vi "AcquisitionFastMode.vi"(10 "Data In":T1={"DAQ Config Data"={"Vertical"={"Coupling"=1, "Offset (V)"=-0.5, "Range (V)"=2.0, "Impedance"=50.0}, "Horizontal"={"Offset Time"=0.0, "Sample Time (S)"=22.0, "Sample Points"=1000}, "Trigger\n"={"Lower Level (V)"=-0.02, "Trigger Slope"=1, "Trigger Source"=10}, "Acquisition"={"Trigger Mode"=1, "Initiate Continuously"=0, "Acquire Type"=0, "Acquire Count"=0}, "Channel"=0, "Instrument Handle"=0, "Error"={"status"=FALSE, "code"=0, "source"=""}, "State"=1}, "Acquisition"={"Current"={"Acquiring Now?"=FALSE, "Waveforms Acquired"=0.0, "Start of Acquisition"=timestamp(0 s since 1904-01-01), "Acquisition Name"=""}, "Stop Condition"={"Quota"=3000.0, "Duration (S)"=22, "Stop Condition"=FALSE}, "Config Needed"=FALSE}, "Measurement"={"Waveform"={"t0"=timestamp(0 s since 1904-01-01), "dt"=1.0, "Y"=[]}, "Peak Heights"=[], "Acquisition Time"=timestamp(0 s since 1904-01-01), "File Path"=path "", "TDMS File Handle"=refnum}, "UI References"={"Acquire"=refnum, "Configure DAQ"=refnum, "Measurement (Ch1)"=refnum, "Update Needed?"=FALSE, "New Run"=refnum, "Signal"=refnum}, "Run Info"={"Active Run?"=FALSE, "Run Notes"="Enter in notes explaining the purpose of the run and any unusual steps taken in the process. This should make it clear why the data was taken. e.g. \"Measuring LXe scintillation light with Teflon\" or \"Measuring dark pulses to determine SPE gain.\" Concise is good but precise is better.", "User Name"="", "Campaign ID#"="", "Run Name"="", "Start Time"=timestamp(0 s since 1904-01-01), "End Time"=timestamp(0 s since 1904-01-01)}, "System Status"={"Bias Voltage"=0.0, "SiPM Temperature"=[], "Slow Control User"="", "LXe"=0.0}, "Acquisition Info"={"Trigger Mode"=FALSE, "Acquisition Mode"=FALSE, "Bias Voltage (V)"=0.0, "Preamplifier"=0, "Shaping Amplifier"=0, "Acquisition Notes"="", "1"=FALSE, "2"=FALSE}} {"Acquisition Info"."Shaping Amplifier" items=["CR-200-100ns", "CR-200-1us"]; "Acquisition Info"."Preamplifier" items=["CR-Z-113-1k", "CR-Z-113-5k", "CR-Z-SiPM"]; "DAQ Config Data"."State" items=["Enable"=1, "Disable"=0]; "DAQ Config Data"."Channel" items=["Input Channel 1", "Input Channel 2", "Input Channel 3", "Input Channel 4"]; "DAQ Config Data"."Acquisition"."Acquire Type" items=["Normal"=0, "Average"=1, "Envelope"=2, "Peak Detect"=3, "High Resolution"=4, "Fast"=5, "Equivalent Time"=16]; "DAQ Config Data"."Acquisition"."Initiate Continuously" items=["Continuously"=1, "Single Capture"=0]; "DAQ Config Data"."Acquisition"."Trigger Mode" items=["Auto", "Normal"]; "DAQ Config Data"."Trigger"."Trigger Source" items=["TTL0", "TTL1", "TTL2", "TTL3", "TTL4", "TTL5", "TTL6", "TTL7", "ECL0", "ECL1", "Input Channel 1", "Input Channel 2", "Input Channel 3", "Input Channel 4", "External Trigger Source", "STAR", "Manual Trigger", "Pattern"]; "DAQ Config Data"."Trigger"."Trigger Slope" items=["Rising Edge", "Falling Edge"]; "DAQ Config Data"."Horizontal"."Sample Time (S)" items=["0.5"=0.5, "0.4"=0.4, "0.25"=0.25, "0.2"=0.2, "0.1"=0.1, "0.05"=0.05, "0.04"=0.04, "0.025"=0.025, "0.02"=0.02, "0.01"=0.01, "0.005"=0.005, "0.004"=0.004, "0.0025"=0.0025, "0.002"=0.002, "0.001"=0.001, "5E-4"=0.0005, "4E-4"=0.0004, "2.5E-4"=0.00025, "2E-4"=0.0002, "1E-4"=0.0001, "5E-5"=5e-05, "4E-5"=4e-05, "2E-5"=2e-05, "5E-6"=5e-06, "1E-6"=1e-06, "5E-7"=5e-07, "1E-7"=1e-07, "5E-8"=5e-08, "1E-8"=1e-08]; "DAQ Config Data"."Vertical"."Impedance" items=["50 Ohm"=50.0, "1 MOhm"=1000000.0]; "DAQ Config Data"."Vertical"."Range (V)" items=["10"=10.0, "5"=5.0, "2"=2.0, "1"=1.0, "0.4"=0.4, "0.2"=0.2, "0.08"=0.08, "0.04"=0.04, "0.02"=0.02, "0.01"=0.01]; "DAQ Config Data"."Vertical"."Coupling" items=["AC", "DC"]}) -> (3 "Data Out":T1={"DAQ Config Data"={"Vertical"={"Coupling"=1, "Offset (V)"=-0.5, "Range (V)"=2.0, "Impedance"=50.0}, "Horizontal"={"Offset Time"=0.0, "Sample Time (S)"=22.0, "Sample Points"=1000}, "Trigger\n"={"Lower Level (V)"=-0.02, "Trigger Slope"=1, "Trigger Source"=10}, "Acquisition"={"Trigger Mode"=1, "Initiate Continuously"=0, "Acquire Type"=0, "Acquire Count"=0}, "Channel"=0, "Instrument Handle"=0, "Error"={"status"=FALSE, "code"=0, "source"=""}, "State"=1}, "Acquisition"={"Current"={"Acquiring Now?"=FALSE, "Waveforms Acquired"=0.0, "Start of Acquisition"=timestamp(0 s since 1904-01-01), "Acquisition Name"=""}, "Stop Condition"={"Quota"=3000.0, "Duration (S)"=22, "Stop Condition"=FALSE}, "Config Needed"=FALSE}, "Measurement"={"Waveform"={"t0"=timestamp(0 s since 1904-01-01), "dt"=1.0, "Y"=[]}, "Peak Heights"=[], "Acquisition Time"=timestamp(0 s since 1904-01-01), "File Path"=path "", "TDMS File Handle"=refnum}, "UI References"={"Acquire"=refnum, "Configure DAQ"=refnum, "Measurement (Ch1)"=refnum, "Update Needed?"=FALSE, "New Run"=refnum, "Signal"=refnum}, "Run Info"={"Active Run?"=FALSE, "Run Notes"="Enter in notes explaining the purpose of the run and any unusual steps taken in the process. This should make it clear why the data was taken. e.g. \"Measuring LXe scintillation light with Teflon\" or \"Measuring dark pulses to determine SPE gain.\" Concise is good but precise is better.", "User Name"="", "Campaign ID#"="", "Run Name"="", "Start Time"=timestamp(0 s since 1904-01-01), "End Time"=timestamp(0 s since 1904-01-01)}, "System Status"={"Bias Voltage"=0.0, "SiPM Temperature"=[], "Slow Control User"="", "LXe"=0.0}, "Acquisition Info"={"Trigger Mode"=FALSE, "Acquisition Mode"=FALSE, "Bias Voltage (V)"=0.0, "Preamplifier"=0, "Shaping Amplifier"=0, "Acquisition Notes"="", "1"=FALSE, "2"=FALSE}} {"Acquisition Info"."Shaping Amplifier" items=["CR-200-100ns", "CR-200-1us"]; "Acquisition Info"."Preamplifier" items=["CR-Z-113-1k", "CR-Z-113-5k", "CR-Z-SiPM"]; "DAQ Config Data"."State" items=["Enable"=1, "Disable"=0]; "DAQ Config Data"."Channel" items=["Input Channel 1", "Input Channel 2", "Input Channel 3", "Input Channel 4"]; "DAQ Config Data"."Acquisition"."Acquire Type" items=["Normal"=0, "Average"=1, "Envelope"=2, "Peak Detect"=3, "High Resolution"=4, "Fast"=5, "Equivalent Time"=16]; "DAQ Config Data"."Acquisition"."Initiate Continuously" items=["Continuously"=1, "Single Capture"=0]; "DAQ Config Data"."Acquisition"."Trigger Mode" items=["Auto", "Normal"]; "DAQ Config Data"."Trigger"."Trigger Source" items=["TTL0", "TTL1", "TTL2", "TTL3", "TTL4", "TTL5", "TTL6", "TTL7", "ECL0", "ECL1", "Input Channel 1", "Input Channel 2", "Input Channel 3", "Input Channel 4", "External Trigger Source", "STAR", "Manual Trigger", "Pattern"]; "DAQ Config Data"."Trigger"."Trigger Slope" items=["Rising Edge", "Falling Edge"]; "DAQ Config Data"."Horizontal"."Sample Time (S)" items=["0.5"=0.5, "0.4"=0.4, "0.25"=0.25, "0.2"=0.2, "0.1"=0.1, "0.05"=0.05, "0.04"=0.04, "0.025"=0.025, "0.02"=0.02, "0.01"=0.01, "0.005"=0.005, "0.004"=0.004, "0.0025"=0.0025, "0.002"=0.002, "0.001"=0.001, "5E-4"=0.0005, "4E-4"=0.0004, "2.5E-4"=0.00025, "2E-4"=0.0002, "1E-4"=0.0001, "5E-5"=5e-05, "4E-5"=4e-05, "2E-5"=2e-05, "5E-6"=5e-06, "1E-6"=1e-06, "5E-7"=5e-07, "1E-7"=1e-07, "5E-8"=5e-08, "1E-8"=1e-08]; "DAQ Config Data"."Vertical"."Impedance" items=["50 Ohm"=50.0, "1 MOhm"=1000000.0]; "DAQ Config Data"."Vertical"."Range (V)" items=["10"=10.0, "5"=5.0, "2"=2.0, "1"=1.0, "0.4"=0.4, "0.2"=0.2, "0.08"=0.08, "0.04"=0.04, "0.02"=0.02, "0.01"=0.01]; "DAQ Config Data"."Vertical"."Coupling" items=["AC", "DC"]}, 4 "Waveforms":waveform(dbl)[](array[waveform]))   [LabVIEW 2012]
uses:
  TypeDefs/DataTypes/Data.ctl
  TypeDefs/DataTypes/DAQConfig.ctl
  TypeDefs/DataTypes/Acquisition.ctl
  TypeDefs/DataTypes/Current.ctl
  TypeDefs/DataTypes/StopCondition.ctl
  TypeDefs/DataTypes/Measurement.ctl
  TypeDefs/DataTypes/UIReferences.ctl
  TypeDefs/DataTypes/RunInfo.ctl
  TypeDefs/DataTypes/SystemStatus.ctl
panel:
  # "Shaper Gain"
  # "Self"
  # "Fast"
  # "Solicited"
  # "Standard"
  # "Shaper Gain"
  # "Self"
  # "Fast"
  # "Solicited"
  # "Standard"
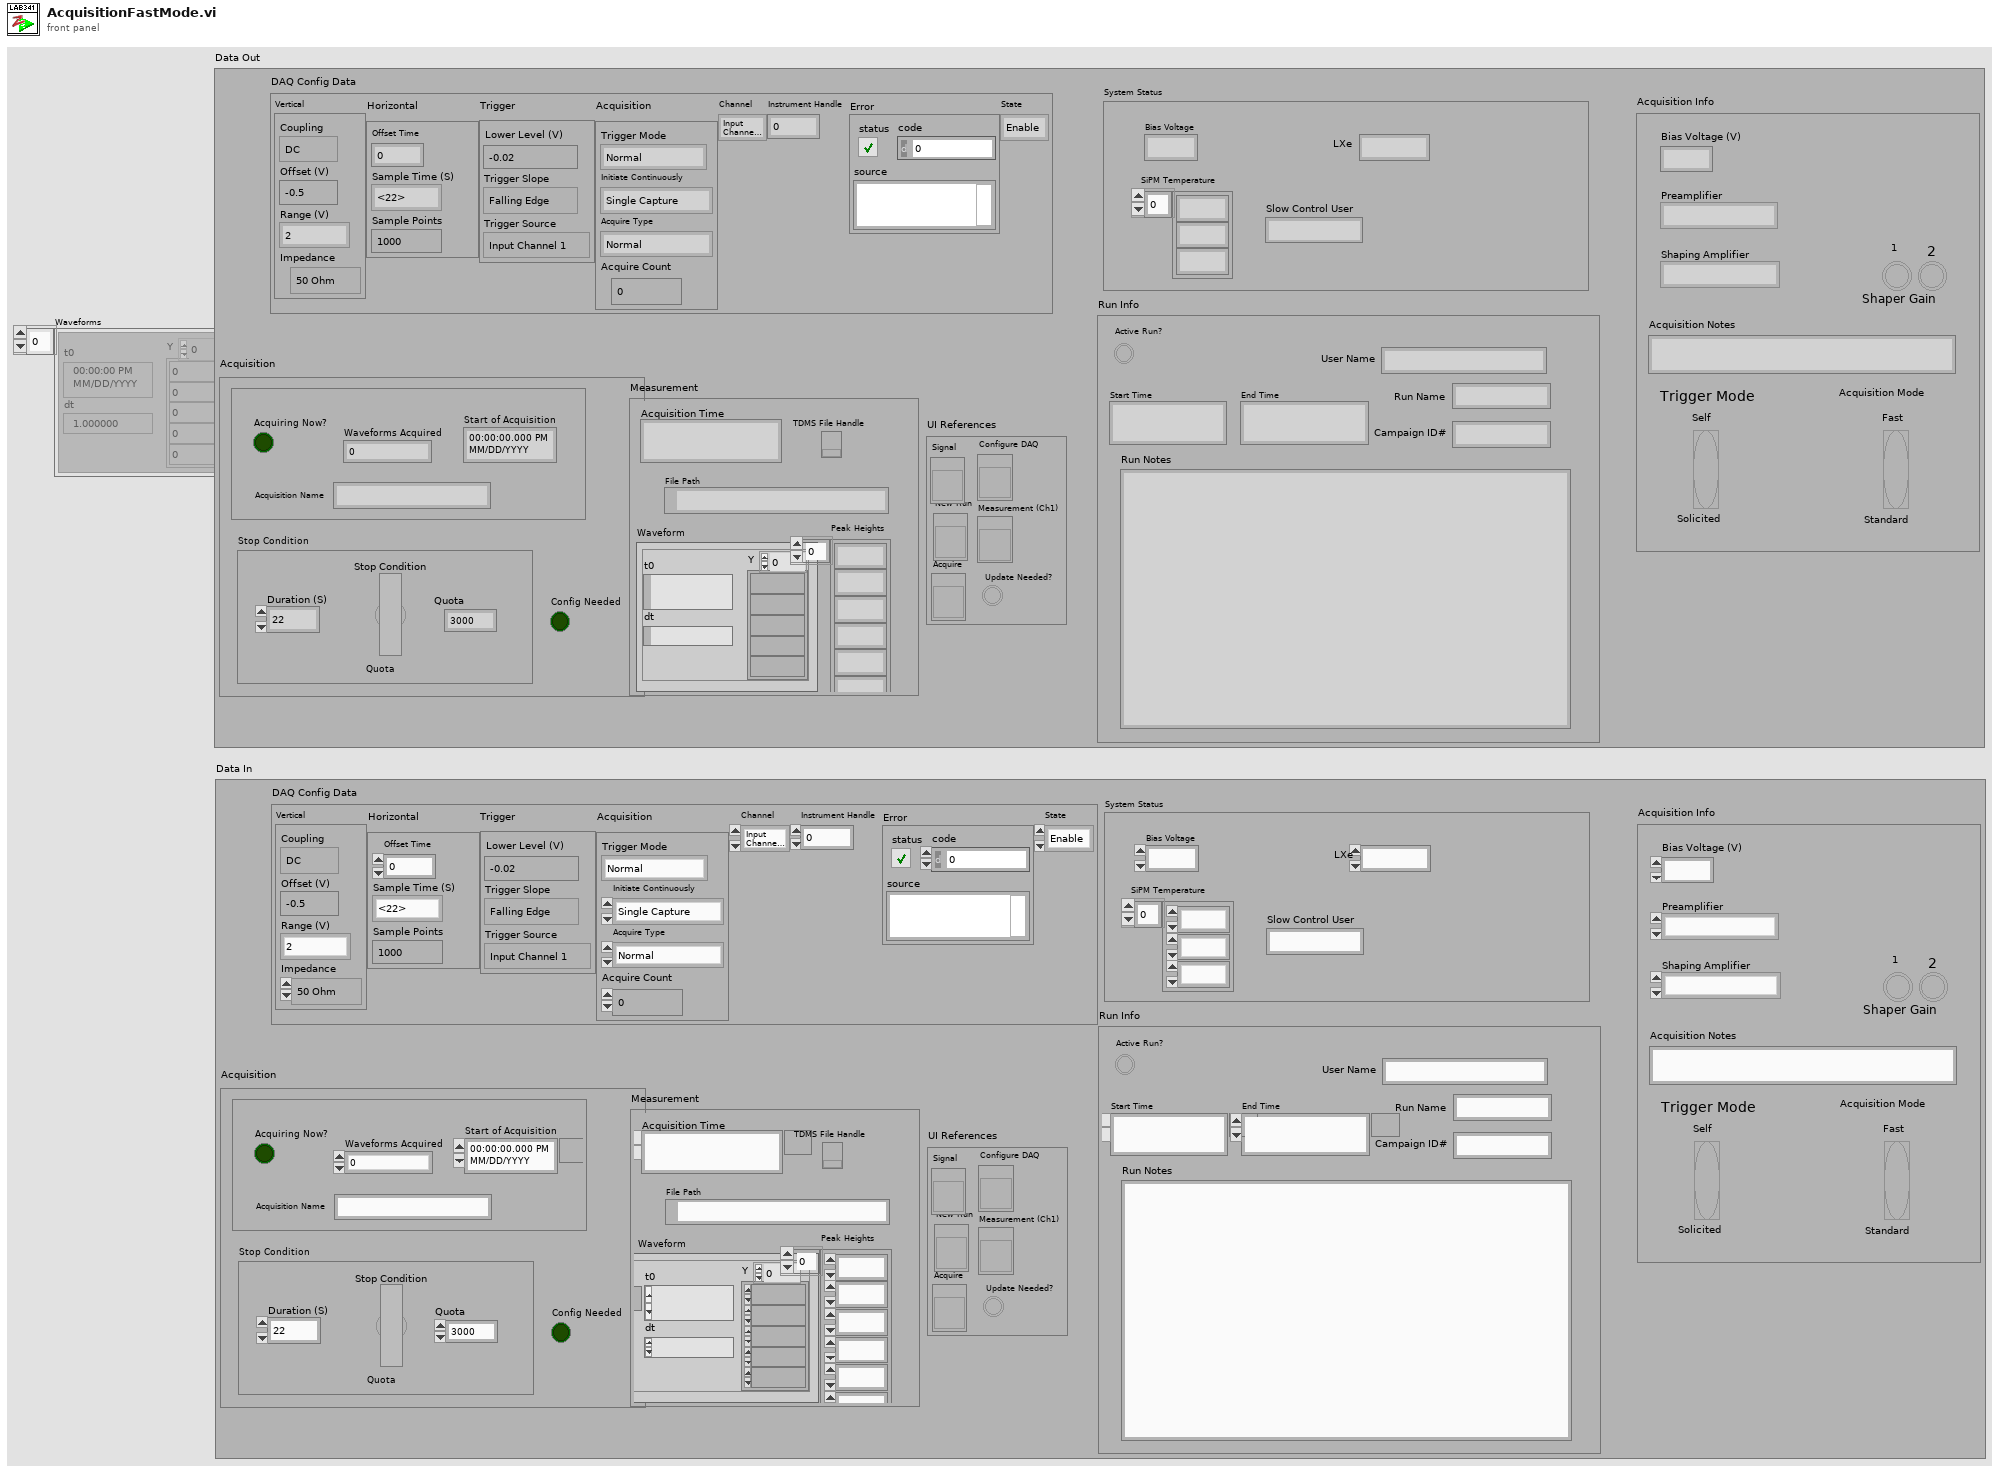
[diagram p1: front panel]
types:
  T1 = typedef "Data.ctl" = cluster{"DAQ Config Data":T2, "Acquisition":T3, "Measurement":T6, "UI References":T7, "Run Info":T8, "System Status":T9, "Acquisition Info":cluster{"Trigger Mode":bool, "Acquisition Mode":bool, "Bias Voltage (V)":dbl, "Preamplifier":u16, "Shaping Amplifier":u16, "Acquisition Notes":string, "1":bool, "2":bool}}
  T2 = typedef "DAQConfig.ctl" = cluster{"Vertical":cluster{"Coupling":i32, "Offset (V)":dbl, "Range (V)":dbl, "Impedance":dbl}, "Horizontal":cluster{"Offset Time":dbl, "Sample Time (S)":dbl, "Sample Points":u32}, "Trigger\n":cluster{"Lower Level (V)":dbl, "Trigger Slope":i32, "Trigger Source":i32}, "Acquisition":cluster{"Trigger Mode":i32, "Initiate Continuously":i32, "Acquire Type":i32, "Acquire Count":i32}, "Channel":i32, "Instrument Handle":i32, "Error":errorcluster, "State":i32}
  T3 = typedef "Acquisition.ctl" = cluster{"Current":T4, "Stop Condition":T5, "Config Needed":bool}
  T4 = typedef "Current.ctl" = cluster{"Acquiring Now?":bool, "Waveforms Acquired":dbl, "Start of Acquisition":timestamp, "Acquisition Name":string}
  T5 = typedef "StopCondition.ctl" = cluster{"Quota":dbl, "Duration (S)":u16, "Stop Condition":bool}
  T6 = typedef "Measurement.ctl" = cluster{"Waveform":waveform(dbl), "Peak Heights":dbl[], "Acquisition Time":timestamp, "File Path":path, "TDMS File Handle":refnum<k34>}
  T7 = typedef "UIReferences.ctl" = cluster{"Acquire":refnum<vi>, "Configure DAQ":refnum<vi>, "Measurement (Ch1)":refnum<vi>, "Update Needed?":bool, "New Run":refnum<vi>, "Signal":refnum<vi>}
  T8 = typedef "RunInfo.ctl" = cluster{"Active Run?":bool, "Run Notes":string, "User Name":string, "Campaign ID#":string, "Run Name":string, "Start Time":timestamp, "End Time":timestamp}
  T9 = typedef "SystemStatus.ctl" = cluster{"Bias Voltage":dbl, "SiPM Temperature":dbl[], "Slow Control User":string, "LXe":dbl}
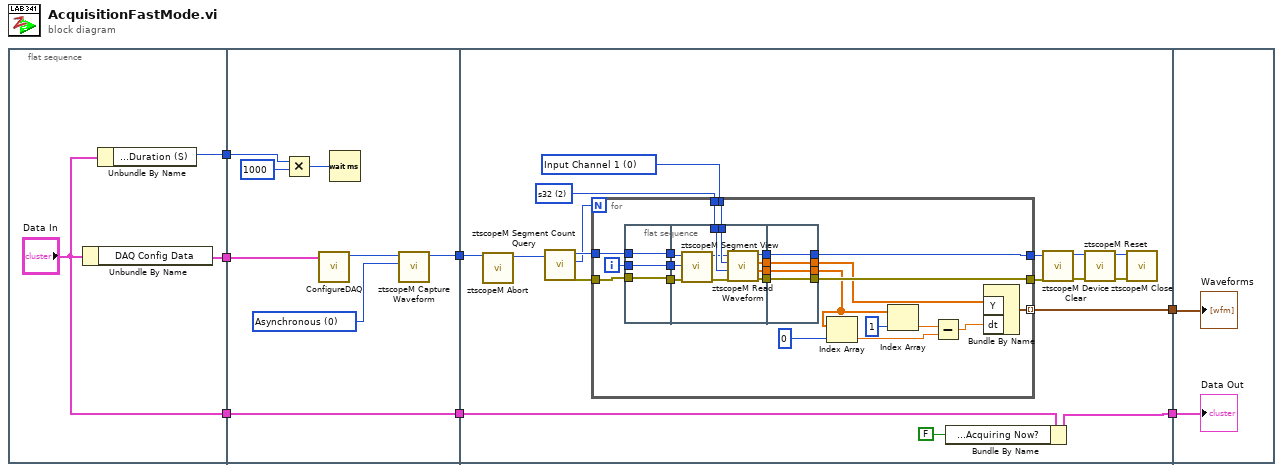
[diagram p0: block diagram]
diagram:
  n1 = flat-sequence {
    tunnel: [w10] -> w5
    tunnel: [w9] -> w4
    tunnel: ["Data In"] -> w1
    tunnel: [w16] -> w6
    tunnel: w5 -> [w15]
    tunnel: w4 -> [w14]
    tunnel: [w11] -> w2
    tunnel: w1 -> [w11]
    tunnel: [w24] -> w7
    tunnel: w6 -> [w23]
    tunnel: [w21] -> w3
    tunnel: w2 -> [w20]
    tunnel: w7 -> [w77]
    tunnel: w3 -> [w76]
    frame #0 {
      n2 = Unbundle By Name("Data In") -> ("DAQ Config Data"=w10:T2)
      n3 = Unbundle By Name("Data In") -> ("Acquisition.Stop Condition.Duration (S)"=w9:u16)
    }
    frame #1 {
      w17 = 0 items=["Infinite"=-1, "Asynchronous"=0] ("Timeout")
      n4 = Multiply(x=w14, y=u16 1000) -> (x*y=w12:u16)
      n5 = call "ConfigureDAQ.vi"("DAQ Config Data"=w15) -> ("Instrument Handle Out"=w18:i32)  [unwired: 9 in, 1 out]
      n6 = Wait (ms)(milliseconds to wait=w12) -> ()  [unwired: 1 out]
      n7 = call <instrlib>:"ztscopeM Capture Waveform.vi"("Timeout"=w17, "Instrument Handle In"=w18) -> ("Instrument Handle Out"=w16:i32)  [unwired: 8 in, 1 out]
    }
    frame #2 {
      w27 = 0 items=["Input Channel 1", "Input Channel 2", "Input Channel 3", "Input Channel 4", "Calc Channel 1", "Calc Channel 2", "Calc Channel 3", "Calc Channel 4", "Ref Channel 1", "Ref Channel 2", "Ref Channel 3", "Ref Channel 4"] ("Source")
      w26 = 2 items=["s8", "s16", "s32", "f32", "f64"] ("Transfer Type")
      n8 = call <instrlib>:"ztscopeM Abort.vi"("Instrument Handle In"=w23) -> ("Instrument Handle Out"=w22:i32)  [unwired: 9 in, 1 out]
      n9 = call <instrlib>:"ztscopeM Segment Count Query.vi"("Instrument Handle In"=w22) -> ("error out"=w30:errorcluster, "Segments"=w25:i32, "Instrument Handle Out"=w31:i32)  [unwired: 8 in]
      n10 = for {
        N: w25 -> [_]
        tunnel: w31 -> [w48]
        tunnel: w30 -> [w50]
        tunnel: w27 -> [w45]
        tunnel: w26 -> [w44]
        tunnel: [w43] -> w29
        tunnel: [w42] -> w28
        tunnel: [w56] -> w24 mode=indexing
        i -> [w47]
        n11 = flat-sequence {
          tunnel: [w60] -> w51
          tunnel: w50 -> [w60]
          tunnel: [w59] -> w49
          tunnel: w48 -> [w59]
          tunnel: w47 -> [w58]
          tunnel: [w58] -> w46
          tunnel: w51 -> [w70]
          tunnel: w49 -> [w64]
          tunnel: w46 -> [w69]
          tunnel: w45 -> [w68]
          tunnel: w44 -> [w67]
          tunnel: [w66] -> w39
          tunnel: [w63] -> w38
          tunnel: [w62] -> w37
          tunnel: [w61] -> w36
          tunnel: [w72] -> w40
          tunnel: [w73] -> w41
          tunnel: [w74] -> w42
          tunnel: [w75] -> w43
          tunnel: w39 -> [w75]
          tunnel: w38 -> [w74]
          tunnel: w37 -> [w73]
          tunnel: w36 -> [w72]
          frame #0 {
          }
          frame #1 {
            n12 = call <instrlib>:"ztscopeM Segment View.vi"("error in"=w70, "Segment Number"=w69, "Instrument Handle In"=w64) -> ("error out"=w71:errorcluster, "Instrument Handle Out"=w65:i32)  [unwired: 7 in]
            n13 = call <instrlib>:"ztscopeM Read Waveform.vi"("error in"=w71, "Transfer Type"=w67, "Source"=w68, "Instrument Handle In"=w65) -> ("error out"=w63:errorcluster, "Time"=w62:dbl[], "Waveform"=w61:dbl[], "Instrument Handle Out"=w66:i32)  [unwired: 4 in]
          }
          frame #2 {
          }
        }
        n14 = Index Array(array=w41, index=0) -> (element=w53:dbl)
        n15 = Index Array(array=w41, index=1) -> (element=w54:dbl)
        n16 = Subtract(x=w54, y=w53) -> (x-y=w52:dbl)
        n17 = Bundle By Name("Y"=w40, "dt"=w52) -> (w56:waveform(dbl))  [unwired: 1 in]
      }
      n18 = Bundle By Name(cluster=w20, "Acquisition.Current.Acquiring Now?"=FALSE) -> (w21:T1)
      n19 = call <instrlib>:"ztscopeM Device Clear.vi"("error in"=w28, "Instrument Handle In"=w29) -> ("error out"=w33:errorcluster, "Instrument Handle Out"=w35:i32)  [unwired: 8 in]
      n20 = call <instrlib>:"ztscopeM Reset.vi"("error in"=w33, "Instrument Handle In"=w35) -> ("error out"=w34:errorcluster, "Instrument Handle Out"=w32:i32)  [unwired: 8 in]
      n21 = call <instrlib>:"ztscopeM Close.vi"("error in"=w34, "Instrument Handle In"=w32) -> ()  [unwired: 9 in, 1 out]
    }
    frame #3 {
      "Waveforms" <- w77
      "Data Out" <- w76
    }
  }
